vi "ICNC Ext SPI Control.vi"(8 "error in (no error)":errorcluster caption="entrée d'erreur (pas d'erreur)", 9 "ReceiveptBuffer":string, 10 "SendptBuffer":string, 11 "SendByteCount":i32) -> (0 "error out":errorcluster caption="sortie d'erreur", 1 "ReceiveptBuffer out":string, 2 "SendptBuffer out":string, 3 "function return":u32)   [LabVIEW 2012, in "ICNC2.lvlib"]
doc: "DWORD ICNC_ExtSPIControl ( int SendByteCount,\n unsigned char *SendptBuffer,\n unsigned char *ReceiveptBuffer) ;"
uses:
  <userlib>/ICNC/ICNC2.lvlib
  <userlib>/ICNC/ICNC2.dll
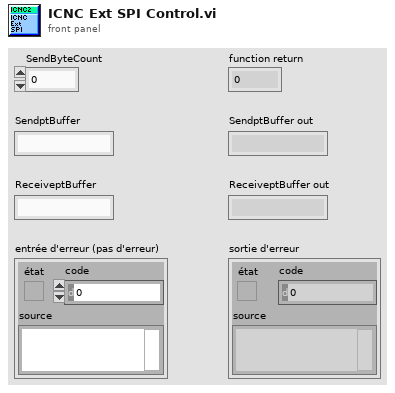
[diagram p1: front panel]
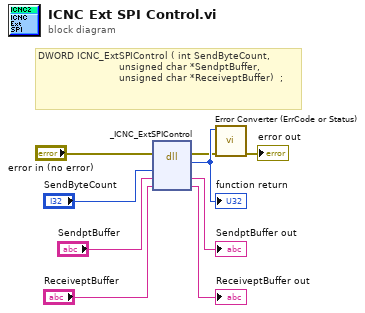
[diagram p0: block diagram]
diagram:
  # "DWORD ICNC_ExtSPIControl ( int SendByteCount,\n                           unsigned char *SendptBuffer,\n                           unsigned char *ReceiveptBuffer)  ;"
  n1 = dll-call lib="C:/Program Files (x86)/National Instruments/LabVIEW 2012/user.lib/ICNC/ICNC2.*" fn="_ICNC_ExtSPIControl"(error in="error in (no error)", "SendByteCount"="SendByteCount", "SendptBuffer"="SendptBuffer", "ReceiveptBuffer"="ReceiveptBuffer") -> (error out=w2:errorcluster, w9:u32, "SendptBuffer"=→"SendptBuffer out":string, "ReceiveptBuffer"=→"ReceiveptBuffer out":string)  [unwired: 3 in, 1 out]
  "function return" <- w9
  n2 = call <userlib>:"Error Converter (ErrCode or Status).vi"("error in (no error)"=w2, "error code"=w9) -> ("error out"=→"error out":errorcluster)  [unwired: 9 in]
